vi "music_reconstruct.vi"() -> ()   [LabVIEW 2026]
uses:
  <vilib>/sound2/lvsound2.llb/Sound Data Format.ctl
panel:
  in  "sound format":T1={"sample rate (S/s)"=22050.0, "number of channels"=2, "bits per sample"=16}
  in  "output bit stream 2":i8[](array[numeric]) caption="output bit stream"
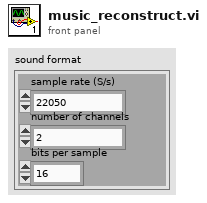
[diagram p1: front panel]
types:
  T1 = typedef "Sound Data Format.ctl" = cluster{"sample rate (S/s)":dbl, "number of channels":i32, "bits per sample":i32}
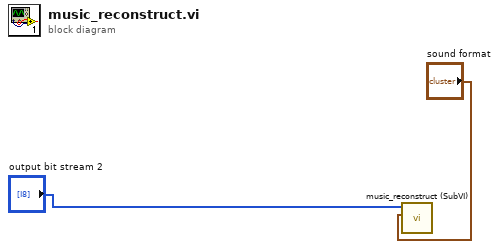
[diagram p0: block diagram]
diagram:
  n1 = call "music_reconstruct (SubVI).vi"("sound format"="sound format", "output bit stream in"="output bit stream 2") -> ()  [unwired: 10 in]
